vi "Get Execution Ref.vi"(8 "error in (no error)":errorcluster, 11 "Execution in":refnum<class "Execution.lvclass">) -> (0 "error out":errorcluster, 2 "Execution Ref":refnum<k7>, 3 "Execution out":refnum<class "Execution.lvclass">)   [LabVIEW 2020, in "TSnax.lvlib" / "Execution.lvclass"]
uses:
  Execution.lvclass
  Execution.lvclass/Execution.ctl
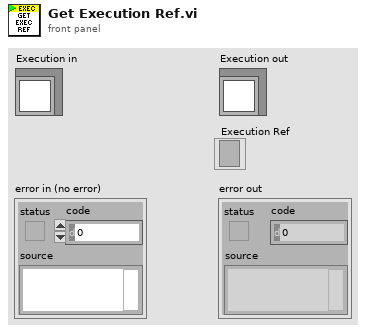
[diagram p1: front panel]
types:
  T1 = typedef "TSnax.lvlib/Execution.lvclass/Ref Data.ctl" = cluster{"Parameters":refnum<class "PropertyObject.lvclass">, "Client Sequence":refnum<class "SequenceFile.lvclass">, "Process Model":refnum<class "SequenceFile.lvclass">, "Entry Sequence":string, "Execution":refnum<k7>, "Report":refnum<class "Report.lvclass">, "Options":T2}
  T2 = typedef "TSnax.lvlib/Execution.lvclass/Execution Options.ctl" = cluster{"Use Default Model":bool, "Release Related Sessions":bool}
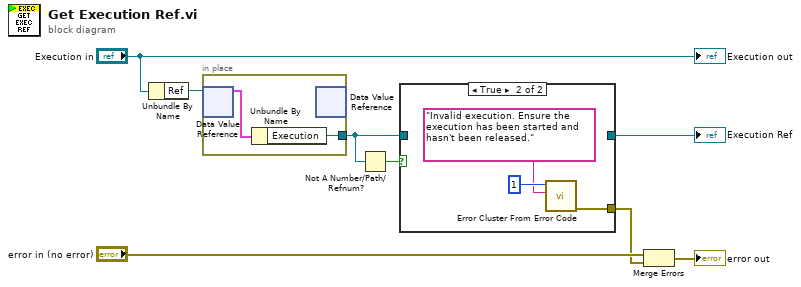
[diagram p0: block diagram]
diagram:
  n1 = Unbundle By Name("Execution in") -> ("Ref"=w7:refnum<data-value>)
  n2 = in-place {
    in-place-border: [w9] -> w4
    n3 = in-place-dvr #1(w7) -> (w10:T1)  [unwired: 1 out]
    n4 = Unbundle By Name(w10) -> ("Execution"=w9:refnum<k7>)
    n5 = in-place-dvr #1() -> ()  [unwired: 1 in, 2 out]
  }
  n6 = Not A Number/Path/Refnum?(number/path/refnum=w4) -> (NaN/Path/Refnum?=w5:bool)
  n7 = case shown="True" w5 {
    tunnel: w4 -> [w11 _]
    tunnel: [w11 _] -> w3
    tunnel: [_ w12] -> w1
    frame False {
    }
    frame True {
      n8 = call <vilib>:"Error Cluster From Error Code.vi"("error message (\"\")"="Invalid execution. Ensure the execution has been started and hasn't been released." ("error message (\"\")"), "error code (0)"=1) -> ("error out"=w12:errorcluster)  [unwired: 7 in]
    }
  }
  "Execution Ref" <- w3
  n9 = Merge Errors("error in (no error)", w1) -> (→"error out":errorcluster)
  "Execution out" <- "Execution in"
